vi "Stop Core.vi"(10 "final error code":i32, 11 "IDialogBox in":refnum<class "IDialogBox.lvclass">) -> (3 "IDialogBox out":refnum<class "IDialogBox.lvclass">)   [LabVIEW 2017, in "IDialogBox.lvlib" / "IDialogBox.lvclass"]
doc: "(<B>Filename</B>: Actor Framework.lvlib:Actor.lvclass:Stop Core.vi)\n\nDefines what the actor does before it stops. Use the <B>final error code</B> input to determine whether the actor shut down in response to an error.\n\nBy default, this method does nothing. A descendant class may override it to define behavior, such as shutting down any processes the actor initiated in its override of the Actor Core method.\n\n<License>\nCopyright © 2017 Composed Systems, LLC | All rights reserved\nwww.composed.io\n\nAuthor: Ethan Stern <ethan.stern@composed.io>\n\nThis software is provided \"AS IS\" WITHOUT WARRANTIES, either express or implied, AND IS FOR EDUCATIONAL PURPOSES ONLY.\n</License>"
uses:
  IDialogBox.lvclass
  C:/Git/mva-framework/gpm_packages/@cs/mva-viewable/Source/IViewable/IViewable/IViewable.lvclass
  gpm_packages/@cs/mva-viewable/Source/IViewable/IViewable/IViewable.lvclass/IViewable.ctl
  gpm_packages/@cs/mva-viewable/Source/IViewable/IViewable/IViewable.lvclass
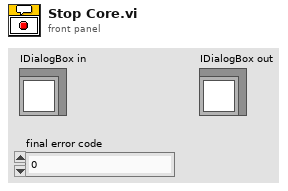
[diagram p1: front panel]
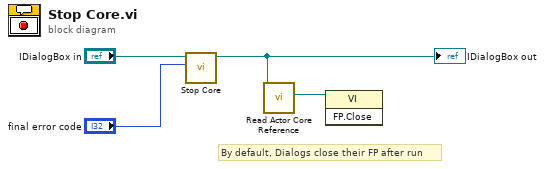
[diagram p0: block diagram]
diagram:
  # "By default, Dialogs close their FP after run"
  n1 = call-parent "Stop Core.vi"("final error code"="final error code", "IViewable in"="IDialogBox in") -> ("IViewable out"=w2:refnum<class "IDialogBox.lvclass">)  [unwired: 9 in]
  "IDialogBox out" <- w2
  n2 = call "Read Actor Core Reference.vi"("IViewable In"=w2) -> ("Actor Core Refnum"=w1:refnum<vi>)  [unwired: 9 in, 1 out]
  n3 = invoke class="VI" method="FP.Close"(reference=w1) -> ()  [unwired: 2 in, 3 out]
